vi "Read Header File.vi"(8 "error in (no error)":errorcluster, 11 "CCD in":refnum<class "CCD.lvclass">) -> (0 "error out":errorcluster, 2 "Header Contents":string[](array[string]), 3 "CCD out":refnum<class "CCD.lvclass">)   [LabVIEW 2018, in "CCD.lvclass"]
uses:
  CCD.lvclass
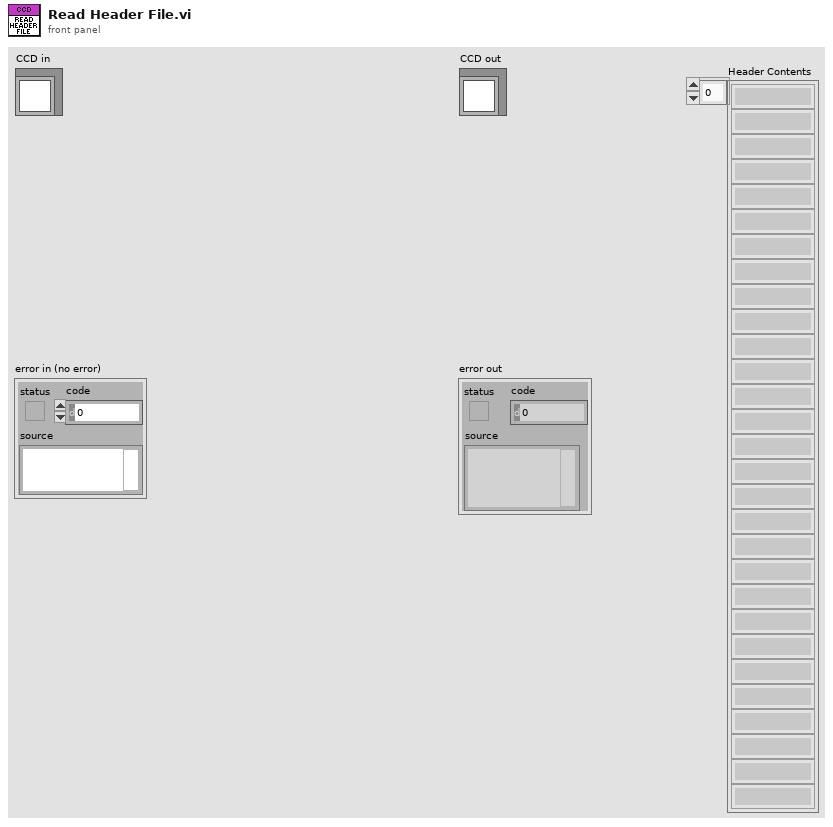
[diagram p1: front panel]
types:
  T1 = enum16{"open", "replace", "create", "open or create", "replace or create", "replace or create with confirmation"}
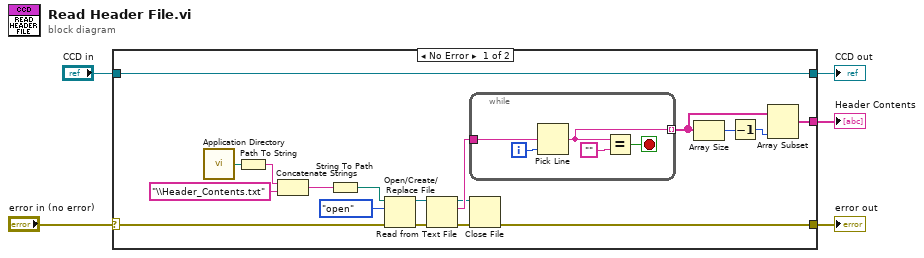
[diagram p0: block diagram]
diagram:
  n1 = case shown="No Error" "error in (no error)" {
    selector: "error in (no error)" -> [w18 w30]
    tunnel: [w15 w30] -> w3
    tunnel: [w10 w29] -> w2
    tunnel: "CCD in" -> [w10 w29]
    tunnel: [w14 _] -> w1
    frame No Error {
      n2 = call <vilib>:"Application Directory.vi"() -> ("Application Directory"=w6:path)
      n3 = Path To String(path=w6) -> (string=w7:string)
      n4 = Concatenate Strings(w7, "\\Header_Contents.txt") -> (w8:string)
      n5 = String To Path(string=w8) -> (path=w19:path)
      n6 = Open/Create/Replace File(file path (use dialog)=w19, error in=w18, operation (0:open)=T1."open") -> (refnum out=w21:refnum<file>, error out=w22:errorcluster)  [unwired: 3 in, 1 out]
      n7 = Read from Text File(file (use dialog)=w21, error in=w22) -> (refnum out=w16:refnum<file>, text=w20:string, error out=w17:errorcluster)  [unwired: 2 in, 1 out]
      n8 = while {
        tunnel: w20 -> [w28]
        tunnel: [w24] -> w13 mode=indexing
        i -> [w27]
        stop <- w25 stop-if-true
        n9 = Pick Line(multi-line string=w28, line index=w27) -> (output string=w24:string)  [unwired: 1 in]
        n10 = Equal?(x=w24, y="") -> (x = y?=w25:bool)
      }
      n11 = Close File(refnum=w16, error in=w17) -> (error out=w15:errorcluster)  [unwired: 1 out]
      n12 = Array Size(array=w13) -> (size(s)=w12:i32)
      n13 = Decrement(x=w12) -> (x-1=w11:i32)
      n14 = Array Subset(array=w13, length=w11) -> (w14:string[])  [unwired: 1 in]
    }
    frame Error {
    }
  }
  "error out" <- w3
  "CCD out" <- w2
  "Header Contents" <- w1
